vi "Change Detect String.vi"(1 "In":string) -> (0 "Changed?":bool)   [LabVIEW 2014]
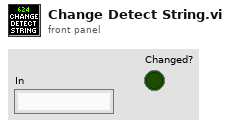
[diagram p1: front panel]
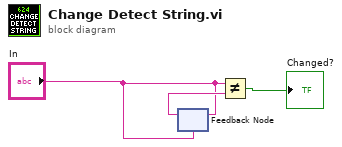
[diagram p0: block diagram]
diagram:
  n1 = feedback-in #1("In") -> ()
  n2 = feedback #1("In") -> (w3:string)
  n3 = Not Equal?(x="In", y=w3) -> (x != y?=→"Changed?":bool)
